vi "test Action Update Ramp Rate-RampRate30.vi"() -> ()   [LabVIEW 2018, in "Action Update Ramp Rate.lvclass"]
uses:
  Action Update Ramp Rate.lvclass
  Libraries/Thermal Chamber Controller_DQMH/Thermal Chamber Controller_DQMH.lvlib
  Libraries/Thermal Chamber Response Simulator/Thermal Chamber Response Simulator.lvlib
panel:
  out "TestCase out":refnum<class "Action Update Ramp Rate.lvclass">
  in  "TestCase in":refnum<class "Action Update Ramp Rate.lvclass">
  out "error out":errorcluster
  in  "error in (no error)":errorcluster
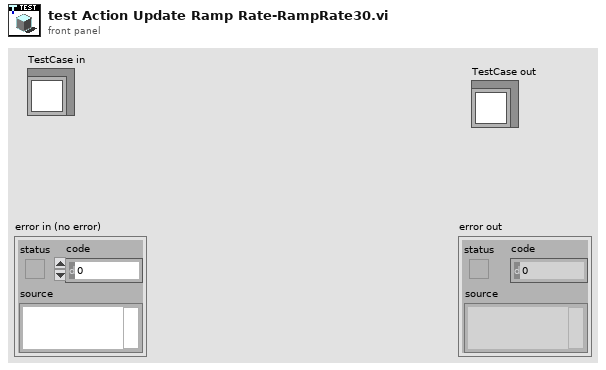
[diagram p1: front panel]
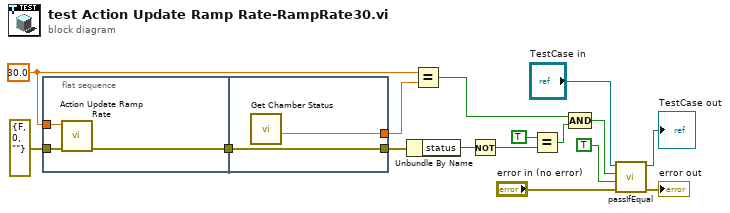
[diagram p0: block diagram]
diagram:
  w3 = 30.0 ("Temperature Set Point")
  n1 = flat-sequence {
    tunnel: errorcluster {"status"=FALSE, "code"=0, "source"=""} ("error in (no error)") -> [w18]
    tunnel: w3 -> [w17]
    tunnel: [w19] -> w5
    tunnel: [w21] -> w8
    tunnel: w5 -> [w21]
    tunnel: [w20] -> w4
    frame #0 {
      n2 = call "Action Update Ramp Rate.vi"("error in (no error)"=w18, "Temperature Ramp Rate"=w17) -> ("error out"=w19:errorcluster)  [unwired: 9 in]
    }
    frame #1 {
      n3 = call "Get Chamber Status.vi"() -> ("Ramp Rate (deg C / second)"=w20:dbl)  [unwired: 6 in, 5 out]
    }
  }
  n4 = Unbundle By Name(w8) -> ("status"=w10:bool)
  n5 = Equal?(x=w3, y=w4) -> (x = y?=w12:bool)
  n6 = Not(x=w10) -> (.not. x?=w9:bool)
  n7 = Equal?(x=TRUE, y=w9) -> (x = y?=w11:bool)
  n8 = Compound Arithmetic op=AND(w12, w11) -> (w7:bool)
  n9 = call-dynamic "passIfEqual.vi"("error in (no error)"="error in (no error)", "y"=TRUE, "x"=w7, "TestCase in"="TestCase in") -> ("error out"=→"error out":errorcluster, "TestCase out"=→"TestCase out":refnum<class "Action Update Ramp Rate.lvclass">)  [unwired: 6 in]
